vi "TX-ADAR-DETECT(LC).vi"(0 "COMPORT":refnum<visa-resource-name>="COM4", 7 "RevC(t)":bool=TRUE, 11 "error in (no error)":errorcluster, 12 "Ant_Sel":i32=1, 13 "Open/Close Serial":bool) -> (3 "string":string="wr txm 0x4A 0x76;wr txm 0x49 0x72", 4 "comport":refnum<visa-resource-name>="COM4", 8 "adc read":dbl=86.0, 15 "error out":errorcluster)   [LabVIEW 2018]
panel:
  out "ADAR":i32=1
  out "Str2":string
  out "Str1":string
  out "number":i32=86
  out "after substring":string="56\r\n>\r\n"
  out "All Success":bool=TRUE
  out "output 2":string="\rwr txm 0x4A 0x76\r\n>\rwr txm 0x49 0x72\r\n>\r\rwr txm 0x4A 0x76\r\n>\rwr txm 0x49 0x72\r\n>\rrd txm 0x4B\r\n0x04B: 0x56\r\n>"
  out "Success":bool[](array[boolean])=[TRUE, TRUE, TRUE, TRUE, TRUE, TRUE]
  # "0 for temperature, 13 for Testport"
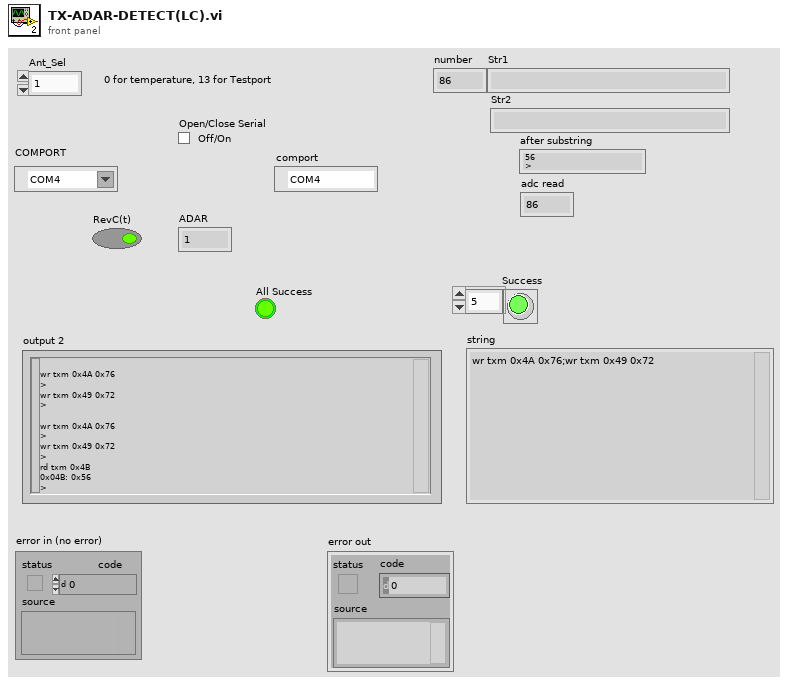
[diagram p1: front panel]
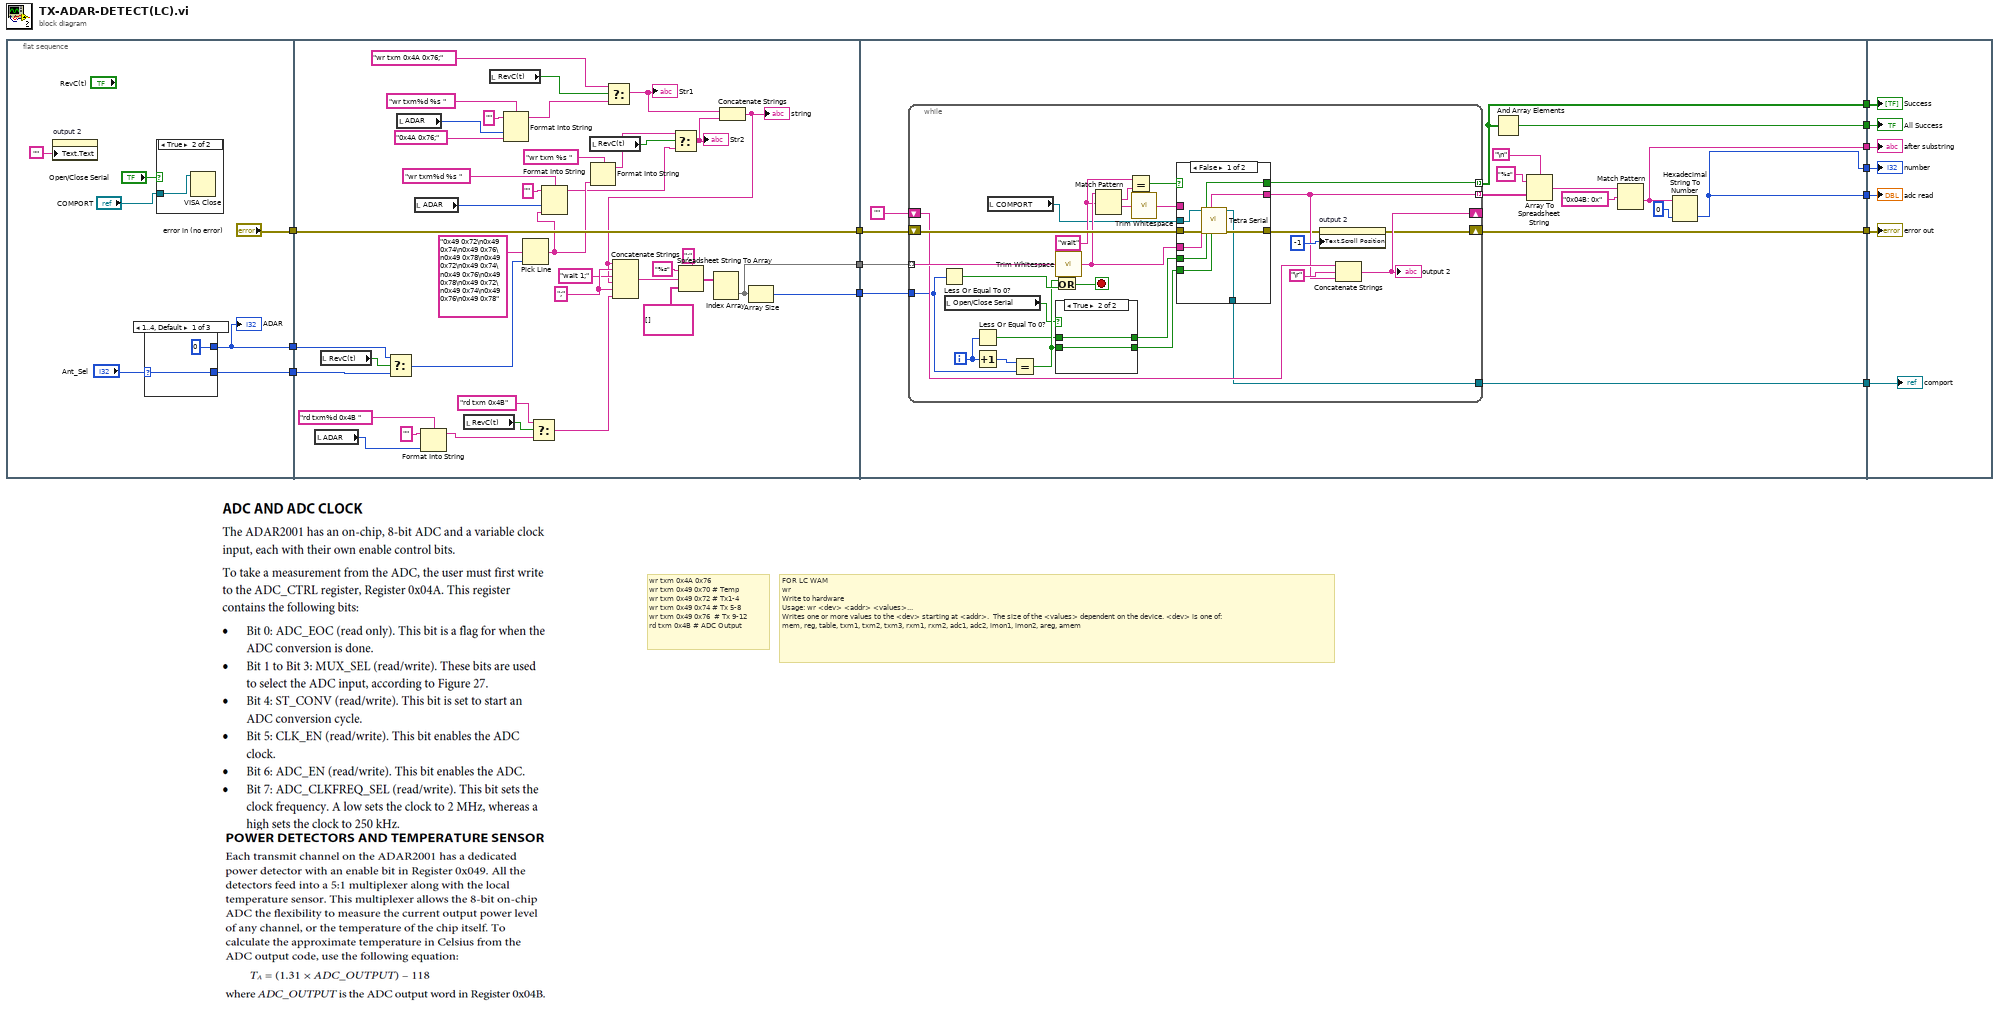
[diagram p0: block diagram]
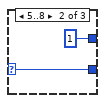
[diagram p2: hidden frame]
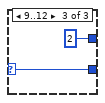
[diagram p3: hidden frame]
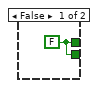
[diagram p5: hidden frame]
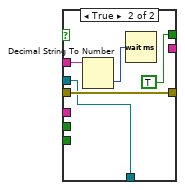
[diagram p6: hidden frame]
diagram:
  # "FOR LC WAM\nwr\nWrite to hardware\nUsage: wr <dev> <addr> <values>...\nWrites one or more values to the <dev> starting at <addr>.  The size of the <values> dependent on the device. <dev> is one of:\nmem, reg, table, txm1, txm2, txm3, rxm1, rxm2, adc1, adc2, imon1, imon2, areg, amem"
  # "wr txm 0x4A 0x76\nwr txm 0x49 0x70 # Temp\nwr txm 0x49 0x72 # Tx1-4\nwr txm 0x49 0x74 # Tx 5-8\nwr txm 0x49 0x76  # Tx 9-12\nrd txm 0x4B # ADC Output"
  n1 = flat-sequence {
    tunnel: ["error in (no error)"] -> w4
    tunnel: [w14] -> w3
    tunnel: [w15] -> w2
    tunnel: [w58] -> w7
    tunnel: [w59] -> w6
    tunnel: [w60] -> w5
    tunnel: w4 -> [w58]
    tunnel: w3 -> [w45]
    tunnel: w2 -> [w48]
    tunnel: [w83] -> w13
    tunnel: [w77] -> w12
    tunnel: [w76] -> w11
    tunnel: [w71] -> w10
    tunnel: [w69] -> w9
    tunnel: [w69] -> w8
    tunnel: w7 -> [w82]
    tunnel: w6 -> [w81]
    tunnel: w5 -> [w74]
    tunnel: [w68] -> w1
    tunnel: w13 -> [w130]
    tunnel: w12 -> [w131]
    tunnel: w11 -> [w132]
    tunnel: w10 -> [w133]
    tunnel: w9 -> [w135]
    tunnel: w8 -> [w134]
    tunnel: w1 -> [w129]
    frame #0 {
      n2 = property on="output 2" class="Str"("Text.Text"="") -> ()  [unwired: 2 in, 2 out]
      n3 = case shown="1..4, Default" "Ant_Sel" {
        selector: "Ant_Sel" -> [w21 w23 w25]
        tunnel: [0 1 2] -> w14
        tunnel: [w21 w23 w25] -> w15
        frame 1..4, Default {
        }
        frame 5..8 {
        }
        frame 9..12 {
        }
      }
      "ADAR" <- w14
      n4 = case shown="True" "Open/Close Serial" {
        tunnel: "COMPORT" -> [_ w27]
        frame False {
        }
        frame True {
          n5 = VISA Close(VISA resource name=w27) -> ()  [unwired: 1 in, 1 out]
        }
      }
    }
    frame #1 {
      w65 = ";" ("string")
      n6 = local read "ADAR"() -> (w29:i32)
      n7 = local read "RevC(t)"() -> (w46:bool)
      n8 = Select(t=w45, s=w46, f=w48) -> (s? t:f=w49:i32)
      n9 = local read "ADAR"() -> (w43:i32)
      n10 = local read "ADAR"() -> (w44:i32)
      n11 = Format Into String(format string="rd txm%d 0x4B " ("multi-line string"), initial string="", w29) -> (resulting string=w28:string)  [unwired: 1 in, 1 out]
      n12 = local read "RevC(t)"() -> (w34:bool)
      n13 = local read "RevC(t)"() -> (w47:bool)
      n14 = Format Into String(format string="wr txm%d %s " ("multi-line string"), initial string="", w43, "0x4A 0x76;" ("Command ( ; seperation)")) -> (resulting string=w52:string)  [unwired: 1 in, 1 out]
      n15 = Pick Line(multi-line string="0x49 0x72\n0x49 0x74\n0x49 0x76\n0x49 0x78\n0x49 0x72\n0x49 0x74\n0x49 0x76\n0x49 0x78\n0x49 0x72\n0x49 0x74\n0x49 0x76\n0x49 0x78", line index=w49) -> (output string=w41:string)  [unwired: 1 in]
      n16 = Select(t="rd txm 0x4B" ("string"), s=w34, f=w28) -> (s? t:f=w32:string)
      n17 = Format Into String(format string="wr txm%d %s " ("multi-line string"), initial string="", w44, w41) -> (resulting string=w39:string)  [unwired: 1 in, 1 out]
      n18 = local read "RevC(t)"() -> (w38:bool)
      n19 = Format Into String(format string="wr txm %s " ("multi-line string"), w41) -> (resulting string=w40:string)  [unwired: 2 in, 1 out]
      n20 = Select(t="wr txm 0x4A 0x76;", s=w47, f=w52) -> (s? t:f=w37:string)
      "Str1" <- w37
      n21 = Select(t=w40, s=w38, f=w39) -> (s? t:f=w36:string)
      "Str2" <- w36
      n22 = Concatenate Strings(w37, w36) -> (w35:string)
      "string" <- w35
      n23 = Concatenate Strings(w35, w65, "wait 1;" ("string"), w35, w65, w32) -> (w67:string)
      n24 = Spreadsheet String To Array(delimiter (Tab)=";", format string="%s", spreadsheet string=w67, array type (2D Dbl)=string[][] []) -> (array=w66:string[][])
      n25 = Index Array(array=w66) -> (element=w59:string[])  [unwired: 2 in]
      n26 = Array Size(array=w59) -> (size(s)=w60:i32)
    }
    frame #2 {
      n27 = while {
        shift-right: [w91] -> w83
        shift-left: w82 -> [w111]
        tunnel: [w106] -> w75 mode=indexing
        tunnel: w81 -> [w110] mode=indexing
        tunnel: w74 -> [w100]
        shift-right: [w104] -> _
        shift-left: "" -> [w107]
        tunnel: [w105] -> w77 mode=indexing
        tunnel: [w84] -> w68
        i -> [w102]
        stop <- w101 stop-if-true
        w94 = "wait" ("regular expression")
        n28 = Less Or Equal To 0?(x=w100) -> (x <= 0?=w99:bool)
        n29 = local read "Open/Close Serial"() -> (w86:bool)
        n30 = Less Or Equal To 0?(x=w102) -> (x <= 0?=w87:bool)
        n31 = Increment(x=w102) -> (x+1=w103:i32)
        n32 = local read "COMPORT"() -> (w85:refnum<visa-resource-name>)
        n33 = Equal?(x=w103, y=w100) -> (x = y?=w90:bool)
        n34 = Or(x=w90, y=w99) -> (x .or. y?=w101:bool)
        n35 = call <vilib>:"Trim Whitespace.vi"("string"=w110) -> ("trimmed string"=w98:string)  [unwired: 1 in]
        n36 = case shown="True" w86 {
          tunnel: w90 -> [_ w114]
          tunnel: [w112 w114] -> w89
          tunnel: [w112 w113] -> w88
          tunnel: w87 -> [_ w113]
          frame False {
            w112 = FALSE
          }
          frame True {
          }
        }
        n37 = Match Pattern(string=w98, regular expression=w94) -> (match substring=w95:string, after substring=w96:string)  [unwired: 1 in, 2 out]
        n38 = Equal?(x=w94, y=w95) -> (x = y?=w97:bool)
        n39 = call <vilib>:"Trim Whitespace.vi"("string"=w96) -> ("trimmed string"=w93:string)  [unwired: 1 in]
        n40 = case shown="False" w97 {
          tunnel: [w123 w126] -> w92
          tunnel: w111 -> [w122 w126]
          tunnel: w88 -> [w121 _]
          tunnel: w89 -> [w120 _]
          tunnel: [w119 _] -> w106
          tunnel: w98 -> [w118 _]
          tunnel: [w117 TRUE ("Success")] -> w105
          tunnel: w85 -> [w116 w124]
          tunnel: w93 -> [_ w128]
          tunnel: [w115 w124] -> w84
          frame False {
            n41 = call "Tetra Serial.vi"("COMPORT"=w116, "error in (no error)"=w122, "Command"=w118, "Open Ser(t)"=w121, "Close Ser(t)"=w120) -> ("Success"=w117:bool, "output"=w119:string, "comport"=w115:refnum<visa-resource-name>, "error out"=w123:errorcluster)  [unwired: 6 in, 1 out]
          }
          frame True {
            n42 = Decimal String To Number(string=w128) -> (number=w127:i32)  [unwired: 2 in, 1 out]
            n43 = Wait (ms)(milliseconds to wait=w127) -> ()  [unwired: 1 out]
          }
        }
        n44 = property on="output 2" class="Str"(error in=w92, "Text.Scroll Position"=-1) -> (error out=w91:errorcluster)  [unwired: 1 in, 1 out]
        n45 = Concatenate Strings(w107, "\r", w106) -> (w104:string)
        "output 2" <- w104
      }
      n46 = And Array Elements(Boolean array=w77) -> (logical AND=w76:bool)
      n47 = Array To Spreadsheet String(delimiter (Tab)="\n", array=w75, 3:"%s" ("format string")) -> (spreadsheet string=w73:string)
      n48 = Match Pattern(string=w73, regular expression="0x04B: 0x") -> (after substring=w71:string)  [unwired: 1 in, 3 out]
      n49 = Hexadecimal String To Number(string=w71, default (0uL)=0 ("default (0 U32)")) -> (number=w69:i32)  [unwired: 1 in, 1 out]
    }
    frame #3 {
      "error out" <- w130
      "comport" <- w129
      "Success" <- w131
      "All Success" <- w132
      "after substring" <- w133
      "adc read" <- w134
      "number" <- w135
    }
  }
